vi "TaDHD.vi"() -> ()   [LabVIEW 2020]
panel:
  in  "HOUR":i32=12 min=-1 max=24 step=1
  out "Actual\ntime":string
  in  "STOP":bool
  in  "DATE":bool
  in  "YEAR":i32=2020 min=2010 max=2070 step=1
  in  "MONTH":i32=6 min=1 max=12 step=1
  in  "DAY":i32=15 min=1 max=31 step=1
  in  "TIME":bool
  in  "MINUTE":i32=30 min=-1 max=60 step=1
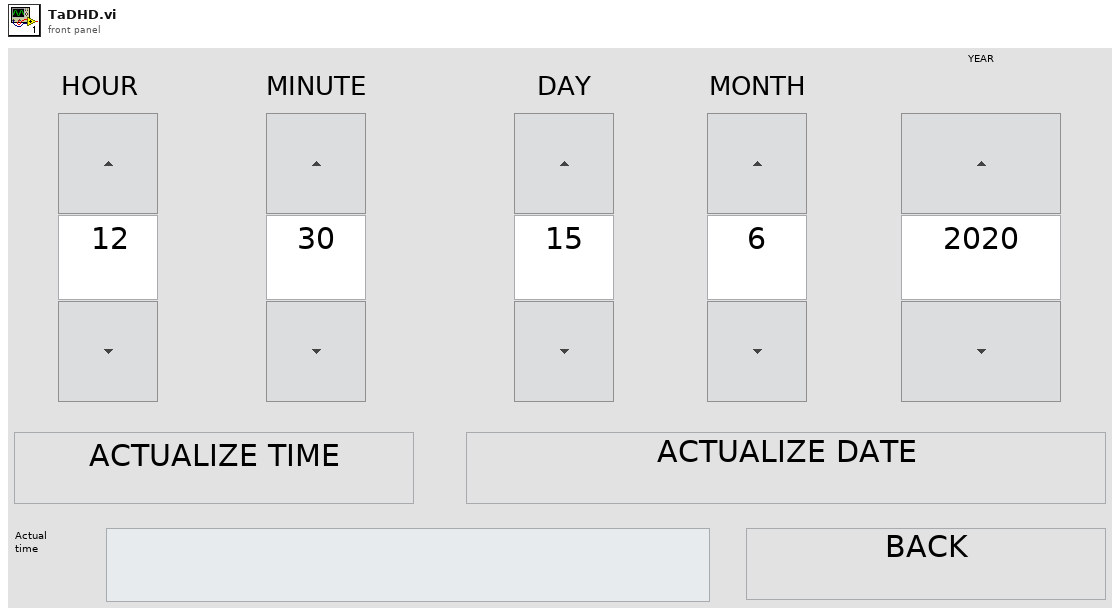
[diagram p1: front panel]
types:
  T1 = enum16{"open", "replace", "create", "open or create", "replace or create", "replace or create with confirmation"}
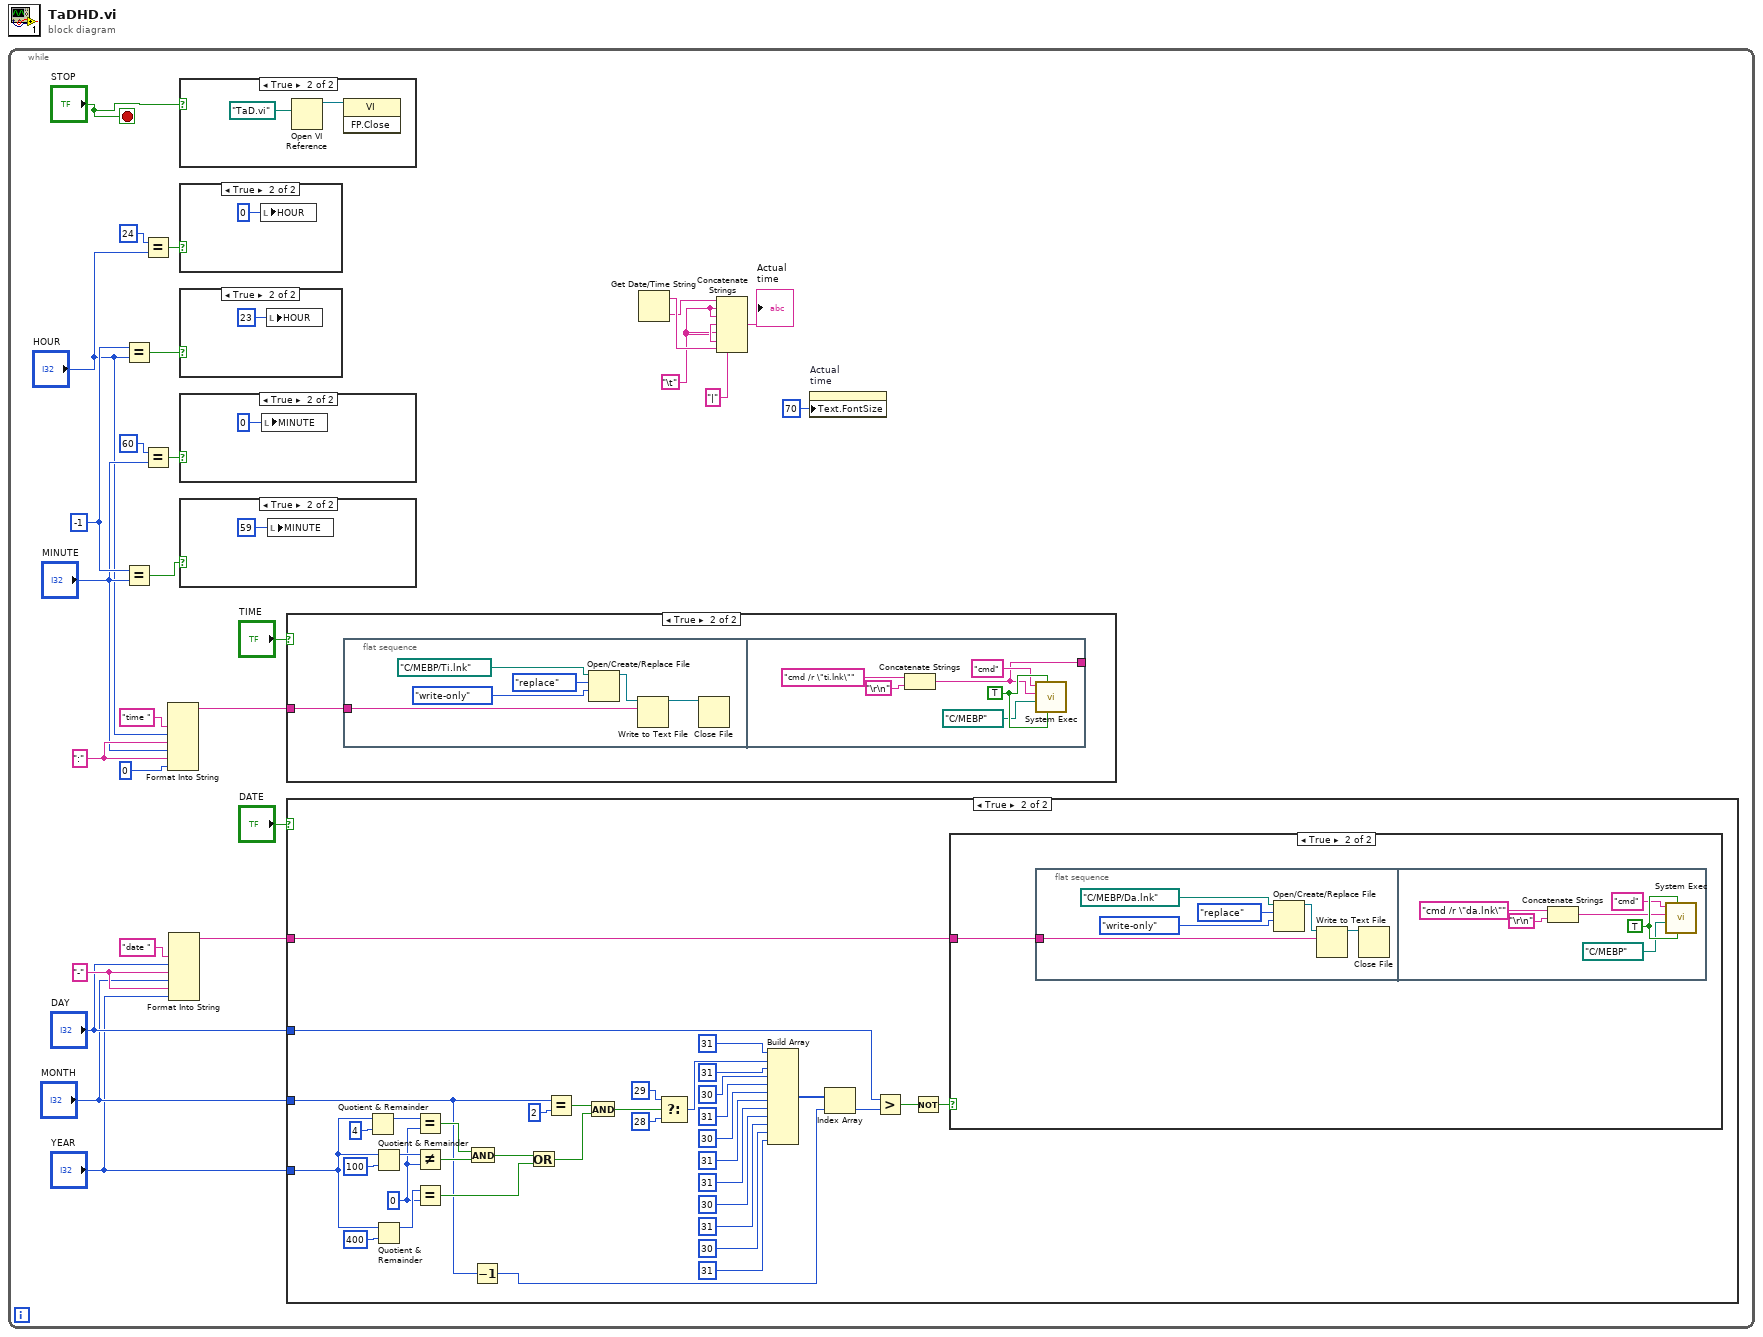
[diagram p0: block diagram]
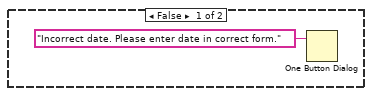
[diagram p4: hidden frame]
diagram:
  n1 = while {
    stop <- "STOP" stop-if-true
    w4 = "\t"
    w15 = "-"
    w25 = -1
    w27 = ":"
    n2 = Equal?(x=w25, y="HOUR") -> (x = y?=w21:bool)
    n3 = Equal?(x=w25, y="MINUTE") -> (x = y?=w20:bool)
    n4 = Equal?(x=24, y="HOUR") -> (x = y?=w22:bool)
    n5 = Equal?(x=60, y="MINUTE") -> (x = y?=w19:bool)
    n6 = Format Into String("time " ("string"), "HOUR", w27, "MINUTE", w27, 0 ("input 6")) -> (resulting string=w13:string)  [unwired: 3 in, 1 out]
    n7 = Format Into String("date " ("string"), "DAY", w15, "MONTH", w15, "YEAR") -> (resulting string=w12:string)  [unwired: 3 in, 1 out]
    n8 = case shown="True" "STOP" {
      frame False {
      }
      frame True {
        n9 = Open VI Reference(vi path=path "TaD.vi") -> (vi reference=w29:refnum<vi>)  [unwired: 5 in, 1 out]
        n10 = invoke class="VI" method="FP.Close"(reference=w29) -> ()  [unwired: 2 in, 3 out]
      }
    }
    n11 = case shown="True" w22 {
      frame False {
      }
      frame True {
        n12 = local write "HOUR"(0 ("Numeric")) -> ()
      }
    }
    n13 = case shown="True" w21 {
      frame False {
      }
      frame True {
        n14 = local write "HOUR"(23 ("Numeric")) -> ()
      }
    }
    n15 = case shown="True" w19 {
      frame False {
      }
      frame True {
        n16 = local write "MINUTE"(0 ("Numeric 2")) -> ()
      }
    }
    n17 = case shown="True" w20 {
      frame False {
      }
      frame True {
        n18 = local write "MINUTE"(59 ("Numeric 2")) -> ()
      }
    }
    n19 = case shown="True" "TIME" {
      tunnel: w13 -> [_ w83]
      frame False {
      }
      frame True {
        n20 = flat-sequence {
          tunnel: w83 -> [w84]
          tunnel: [w90] -> _
          frame #0 {
            n21 = Open/Create/Replace File(file path (use dialog)=path "C:/MEBP/Ti.lnk", operation (0:open)=T1."replace", access (0:read/write)=enum16{"read/write", "read-only", "write-only"}."write-only") -> (refnum out=w88:refnum<file>)  [unwired: 3 in, 2 out]
            n22 = Write to Text File(file (use dialog)=w88, text=w84) -> (refnum out=w89:refnum<file>)  [unwired: 2 in, 2 out]
            n23 = Close File(refnum=w89) -> ()  [unwired: 1 in, 2 out]
          }
          frame #1 {
            w95 = TRUE ("wait until completion? (T)")
            n24 = Concatenate Strings("cmd /r \"ti.lnk\"", "\r\n") -> (w90:string)
            n25 = call <vilib>:"System Exec.vi"("run minimized? (F)"=w95, "wait until completion? (T)"=w95, "working directory"=path "C:/MEBP", "standard input"=w90, "command line"="cmd") -> ()  [unwired: 3 in, 4 out]
          }
        }
      }
    }
    n26 = case shown="True" "DATE" {
      tunnel: w12 -> [_ w54]
      tunnel: "DAY" -> [_ w66]
      tunnel: "MONTH" -> [_ w32]
      tunnel: "YEAR" -> [_ w48]
      frame False {
      }
      frame True {
        w42 = 0 ("y")
        n27 = Quotient & Remainder(x=w48, y=4) -> (x-y*floor(x/y)=w51:i32)  [unwired: 1 out]
        n28 = Quotient & Remainder(x=w48, y=100) -> (x-y*floor(x/y)=w46:i32)  [unwired: 1 out]
        n29 = Quotient & Remainder(x=w48, y=400) -> (x-y*floor(x/y)=w43:i32)  [unwired: 1 out]
        n30 = Equal?(x=w51, y=w42) -> (x = y?=w44:bool)
        n31 = Not Equal?(x=w46, y=w42) -> (x != y?=w45:bool)
        n32 = Equal?(x=w43, y=w42) -> (x = y?=w40:bool)
        n33 = And(x=w44, y=w45) -> (x .and. y?=w41:bool)
        n34 = Decrement(x=w32) -> (x-1=w31:i32)
        n35 = Or(x=w41, y=w40) -> (x .or. y?=w38:bool)
        n36 = Equal?(x=w32, y=2) -> (x = y?=w39:bool)
        n37 = And(x=w39, y=w38) -> (x .and. y?=w37:bool)
        n38 = Select(t=29, s=w37, f=28) -> (s? t:f=w34:i32)
        n39 = Build Array(31, w34, 31, 30, 31, 30, 31, 31, 30, 31, 30, 31) -> (w67:i32[])
        n40 = Index Array(array=w67, index=w31) -> (element=w68:i32)
        n41 = Greater?(x=w66, y=w68) -> (0:w53:bool)
        n42 = Not(x=w53) -> (.not. x?=w33:bool)
        n43 = case shown="True" w33 {
          tunnel: w54 -> [_ w70]
          frame False {
            n44 = One Button Dialog(message="Incorrect date. Please enter date in correct form.") -> ()  [unwired: 1 in, 1 out]
          }
          frame True {
            n45 = flat-sequence {
              tunnel: w70 -> [w71]
              frame #0 {
                n46 = Open/Create/Replace File(file path (use dialog)=path "C:/MEBP/Da.lnk", operation (0:open)=T1."replace", access (0:read/write)=enum16{"read/write", "read-only", "write-only"}."write-only") -> (refnum out=w75:refnum<file>)  [unwired: 3 in, 2 out]
                n47 = Write to Text File(file (use dialog)=w75, text=w71) -> (refnum out=w76:refnum<file>)  [unwired: 2 in, 2 out]
                n48 = Close File(refnum=w76) -> ()  [unwired: 1 in, 2 out]
              }
              frame #1 {
                w82 = TRUE ("wait until completion? (T)")
                n49 = Concatenate Strings("cmd /r \"da.lnk\"", "\r\n") -> (w77:string)
                n50 = call <vilib>:"System Exec.vi"("run minimized? (F)"=w82, "wait until completion? (T)"=w82, "working directory"=path "C:/MEBP", "standard input"=w77, "command line"="cmd") -> ()  [unwired: 3 in, 4 out]
              }
            }
          }
        }
      }
    }
    n51 = Get Date/Time String() -> (date string=w6:string, time string=w5:string)  [unwired: 3 in]
    n52 = Concatenate Strings(w5, w4, w4, "|", w4, w4, w6) -> (→"Actual\ntime":string)
    n53 = property on="Actual\ntime" class="Str"("Text.FontSize"=u32 70 ("Text.Font:Size")) -> ()  [unwired: 2 in, 2 out]
  }
